vi "Day 6 Task 2 attempt 2.vi"() -> ()   [LabVIEW 2018]
panel:
  out "sum":i64
  out "Final fish quantities":i64[](array[numeric])
  out "Initial Fish quantites":i8[](array[numeric])
  out "Fish ages (days)":i32[](array[numeric])
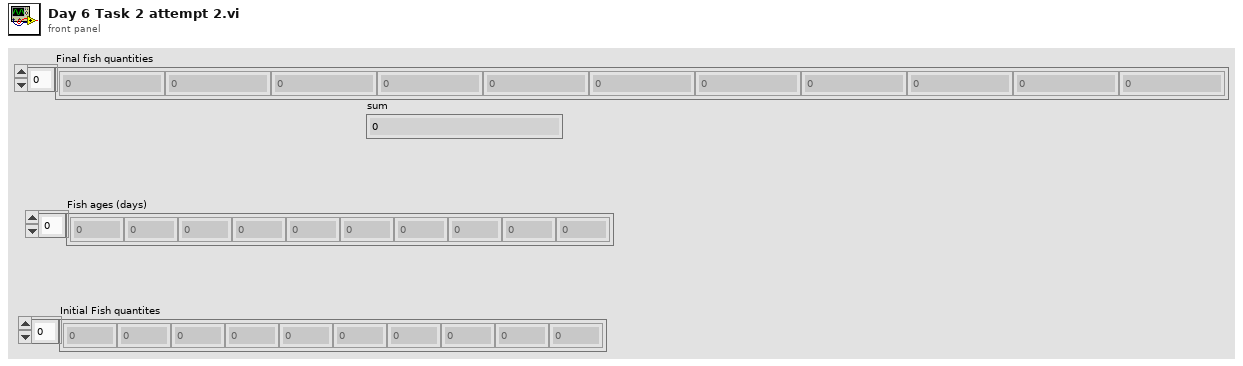
[diagram p1: front panel]
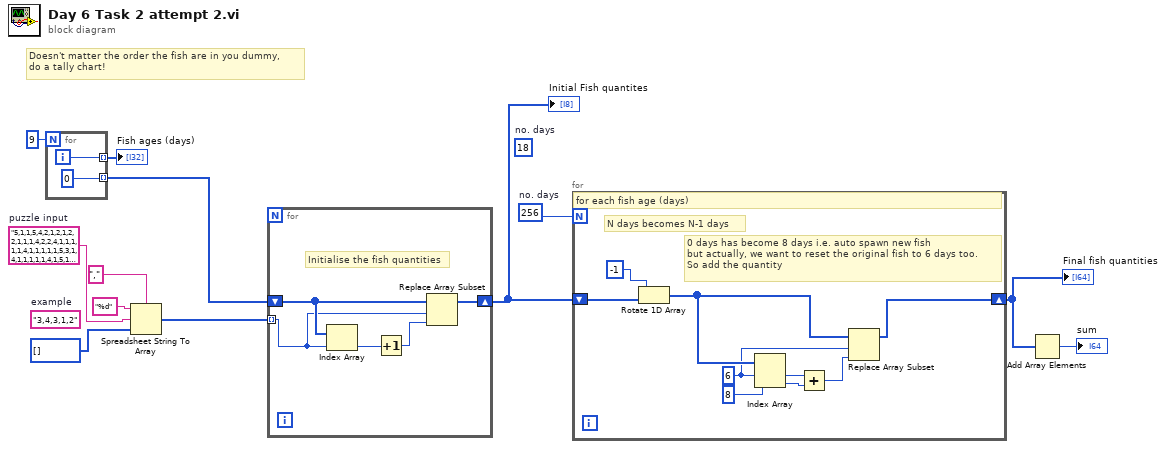
[diagram p0: block diagram]
diagram:
  w1 = "5,1,1,5,4,2,1,2,1,2,2,1,1,1,4,2,2,4,1,1,1,1,1,4,1,1,1,1,1,5,3,1,4,1,1,1,1,1,4,1,5,1,1,1,4,1,2,2,3,1,5,1,1,5,1,1,5,4,1,1,1,4,3,1,1,1,3,1,5,5,1,1,1,1,5,3,2,1,2,3,1,5,1,1,4,1,1,2,1,5,1,1,1,1,5,4,5,1,3,1,3,3,5,5,1,3,1,5,3,1,1,4,2,3,3,1,2,4,1,1,1,1,1,1,1,2,1,1,4,1,3,2,5,2,1,1,1,4,2,1,1,1,4,2,4,1,1,1,1,4,1,3,5,5,1,2,1,3,1,1,4,1,1,1,1,2,1,1,4,2,3,1,1,1,1,1,1,1,4,5,1,1,3,1,1,2,1,1,1,5,1,1,1,1,1,3,2,1,2,4,5,1,5,4,1,1,3,1,1,5,5,1,3,1,1,1,1,4,4,2,1,2,1,1,5,1,1,4,5,1,1,1,1,1,1,1,1,1,1,3,1,1,1,1,1,4,2,1,1,1,2,5,1,4,1,1,1,4,1,1,5,4,4,3,1,1,4,5,1,1,3,5,3,1,2,5,3,4,1,3,5,4,1,3,1,5,1,4,1,1,4,2,1,1,1,3,2,1,1,4"  # puzzle input
  w2 = 256  # no. days
  (unwired) 18  # no. days
  (unwired) "3,4,3,1,2"  # example
  # "Doesn't matter the order the fish are in you dummy,\ndo a tally chart!"
  n1 = for {
    N: 9 -> [_]
    tunnel: [w14] -> w11 mode=indexing
    tunnel: [i64 0] -> w6 mode=indexing
    i -> [w14]
  }
  "Fish ages (days)" <- w11
  n2 = Spreadsheet String To Array(delimiter (Tab)=",", format string="%d", spreadsheet string=w1, array type (2D Dbl)=i64[] []) -> (array=w7:i64[])
  n3 = for {
    tunnel: w7 -> [w18] mode=indexing
    shift-right: [w15] -> w5
    shift-left: w6 -> [w19]
    # "Initialise the fish quantities"
    n4 = Index Array(array=w19, index=w18) -> (element=w16:i64)
    n5 = Increment(x=w16) -> (x+1=w17:i64)
    n6 = Replace Array Subset(array=w19, new element=w17, index=w18) -> (w15:i64[])
  }
  "Initial Fish quantites" <- w5
  n7 = for {
    N: w2 -> [_]
    shift-right: [w24] -> w4
    shift-left: w5 -> [w27]
    w20 = 6 ("index")
    # "0 days has become 8 days i.e. auto spawn new fish\nbut actually, we want to reset the original fish to 6 days too.\nSo add the quantity"
    # "N days becomes N-1 days"
    # "for each fish age (days)"
    n8 = Rotate 1D Array(1:w27, 2:-1 ("n")) -> (0:w25:i64[])
    n9 = Index Array(array=w25, index #1=w20, index #2=8 ("index")) -> (element #1=w21:i64, element #2=w22:i64)
    n10 = Add(x=w21, y=w22) -> (x+y=w23:i64)
    n11 = Replace Array Subset(array=w25, new element=w23, index=w20) -> (w24:i64[])
  }
  "Final fish quantities" <- w4
  n12 = Add Array Elements(numeric array=w4) -> (sum=→"sum":i64)
